vi "6-1.vi"() -> ()   [LabVIEW 2017]
panel:
  out "Waveform Chart 3":dbl(graph)
  out "Waveform Chart 2":dbl(graph)
  in  "stop":bool
  out "Waveform Chart":dbl(graph)
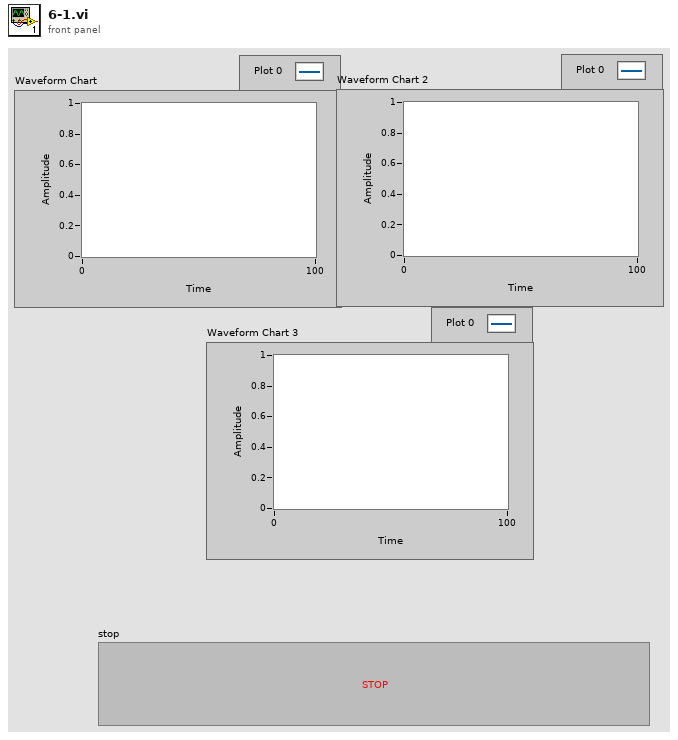
[diagram p1: front panel]
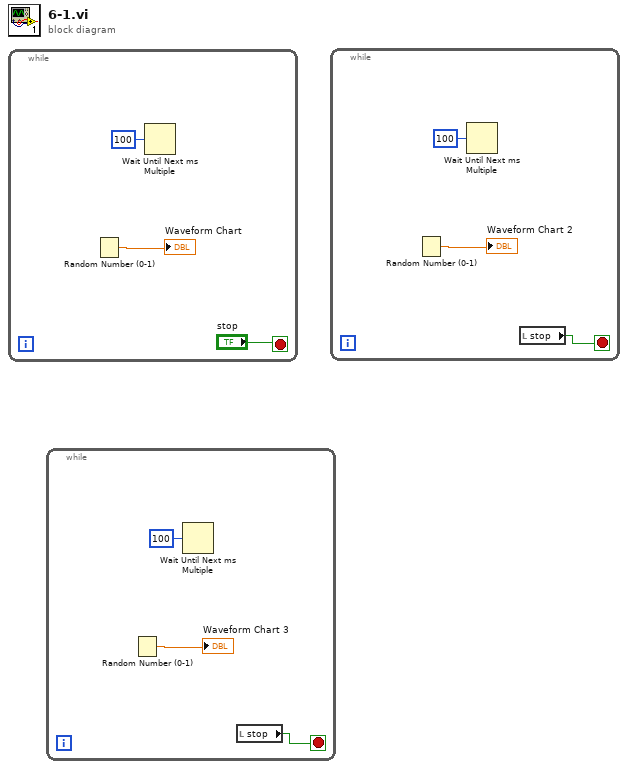
[diagram p0: block diagram]
diagram:
  n1 = while {
    stop <- "stop" stop-if-true
    n2 = Random Number (0-1)() -> (number: 0 to 1=→"Waveform Chart":dbl)
    n3 = Wait Until Next ms Multiple(millisecond multiple=u32 100) -> ()  [unwired: 1 out]
  }
  n4 = while {
    stop <- w4 stop-if-true
    n5 = Random Number (0-1)() -> (number: 0 to 1=→"Waveform Chart 3":dbl)
    n6 = Wait Until Next ms Multiple(millisecond multiple=u32 100) -> ()  [unwired: 1 out]
    n7 = local read "stop"() -> (w4:bool)
  }
  n8 = while {
    stop <- w7 stop-if-true
    n9 = Random Number (0-1)() -> (number: 0 to 1=→"Waveform Chart 2":dbl)
    n10 = Wait Until Next ms Multiple(millisecond multiple=u32 100) -> ()  [unwired: 1 out]
    n11 = local read "stop"() -> (w7:bool)
  }
